vi "five_point_diff_v1.vi"(11 "Signal in (5 point)":dbl[](array[numeric])) -> (3 "dx/dt":dbl)   [LabVIEW 2018]
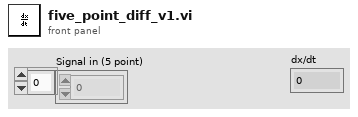
[diagram p1: front panel]
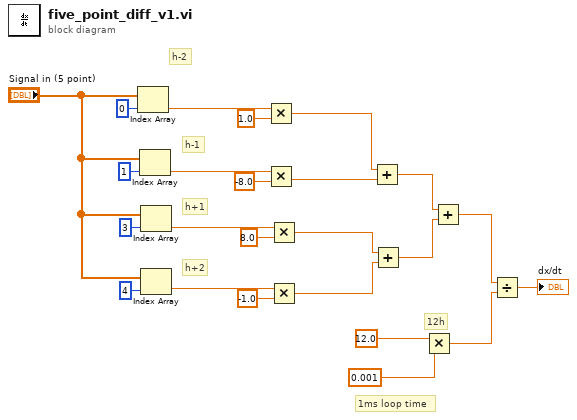
[diagram p0: block diagram]
diagram:
  # "12h"
  # "1ms loop time"
  # "h+2"
  # "h+1"
  # "h-1"
  # "h-2"
  n1 = Index Array "Index Array"(array="Signal in (5 point)", index=0) -> (element=w19:dbl)
  n2 = Index Array(array="Signal in (5 point)", index=1) -> (element=w17:dbl)
  n3 = Index Array(array="Signal in (5 point)", index=3) -> (element=w15:dbl)
  n4 = Index Array(array="Signal in (5 point)", index=4) -> (element=w13:dbl)
  n5 = Multiply(x=w19, y=1.0) -> (x*y=w11:dbl)
  n6 = Multiply(x=w17, y=-8.0) -> (x*y=w10:dbl)
  n7 = Multiply(x=w15, y=8.0) -> (x*y=w9:dbl)
  n8 = Multiply(x=w13, y=-1.0) -> (x*y=w8:dbl)
  n9 = Add(x=w11, y=w10) -> (x+y=w7:dbl)
  n10 = Add(x=w9, y=w8) -> (x+y=w6:dbl)
  n11 = Multiply(x=12.0, y=0.001) -> (x*y=w2:dbl)
  n12 = Add(x=w7, y=w6) -> (x+y=w3:dbl)
  n13 = Divide(x=w3, y=w2) -> (x/y=→"dx/dt":dbl)
